vi "SwissSPAD Live_Refresh All Parameters.vi"(8 "Error In":errorcluster, 9 "Verbose (T)":bool=TRUE, 11 "VI Refnum in":refnum<vi>) -> (0 "Error Out":errorcluster)   [LabVIEW 2021]
uses:
  SwissSPAD Live_Settings List.ctl
  341269f5-52e1-4f88-b524-c1612519b6ae.vi
panel:
  out "Settings Error Source":T1[](array[typedef])
  in  "SS2 Live Settings List":T1
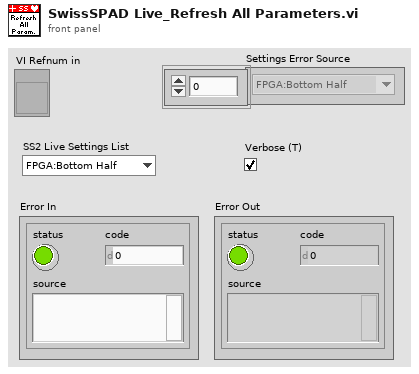
[diagram p1: front panel]
types:
  T1 = typedef "SwissSPAD Live_Settings List.ctl" = enum16{"FPGA:Bottom Half", "FPGA:Top Half", "FPGA:Bottom Bitfile Path", "FPGA:Top Bitfile Path", "FPGA:Bottom Bitstream Version", "FPGA:Top Bitstream Version", "FPGA:Auto Reset FPGA", "FPGA:Bottom FPGA Serial Number", "FPGA:Top FPGA Serial Number", "FPGA:Detector PCB Version", "Acquisition Parameters:Microlens", "Acquisition Parameters:SS2 DAQ Parameters", "Acquisition Parameters:Gate Configuration Array", "Acquisition Parameters:SS3 DAQ Parameters", "Acquisition Parameters:Buffer Size (# 8-bit Gates)", "File Information:File Information", "File Information:# Datasets in Series", "File Information:Scrambled File Flag", "File Information:SS3 Gate Slip Correction", "File Information:SS3 Hot Pixel Mismatch Detection", "File Information:Delay between Datasets", "File Information:Save Sum of All Gates Preview", "Image Parameters:Image ROI Information", "Image Parameters:Image Binning Options", "Image Parameters:SS3 Displayed Image", "Image Parameters:Image Display Options", "Image Parameters:Use Histogram Cursors", "Image Parameter:FPGA Data to Display", "UI Settings:Histogram Bins Number", "UI Settings:Use Image Display Options", "UI Settings:Verbose Settings", "UI Settings:Verbose Saving"}
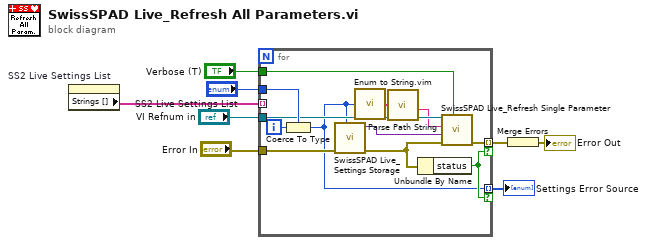
[diagram p0: block diagram]
diagram:
  n1 = property on="SS2 Live Settings List" class="Enum (strict)"() -> ("Strings []"=w6:string[])  [unwired: 2 in, 2 out]
  n2 = for {
    tunnel: "VI Refnum in" -> [w18]
    tunnel: w6 -> [_] mode=indexing
    tunnel: "SS2 Live Settings List" -> [w19]
    tunnel: "Error In" -> [w16]
    tunnel: [w15] -> w4 mode=indexing if=w13
    tunnel: [w10] -> w2 mode=indexing if=w13
    tunnel: "Verbose (T)" -> [w12]
    i -> [w20]
    n3 = Coerce To Type(0:w20, 1:w19) -> (2:w10:T1)
    n4 = call "SwissSPAD Live_Settings Storage.vi"("Settings List"=w10, "Error In"=w16) -> ("Error Out"=w14:errorcluster, "Variant Data out"=w9:variant)  [unwired: 8 in]
    n5 = call "Enum to String.vim"("Enum"=w10) -> ("String"=w11:string)
    n6 = call "Parse Path String.vi"("Path in"=w11) -> ("File/Folder"=w17:string)  [unwired: 4 in, 1 out]
    n7 = Unbundle By Name(w14) -> ("status"=w13:bool)
    n8 = call "SwissSPAD Live_Refresh Single Parameter.vi"("Verbose (T)"=w12, "Error In"=w14, "Data"=w9, "Control Label"=w17, "VI Ref in"=w18) -> ("Error Out"=w15:errorcluster)  [unwired: 6 in]
  }
  "Settings Error Source" <- w2
  n9 = Merge Errors(w4) -> (→"Error Out":errorcluster)
